vi "SetVolume.vi"(0 "reference in":refnum<class "MusicDevice.lvclass">, 2 "Volume":u8 max=100, 5 "Error In":errorcluster) -> (14 "reference out":refnum<class "MusicDevice.lvclass">, 19 "Error Out":errorcluster)   [LabVIEW 2024, in "MusicDevice.lvclass"]
uses:
  MusicDevice.lvclass
  MusicDevice.lvclass/MusicDevice.ctl
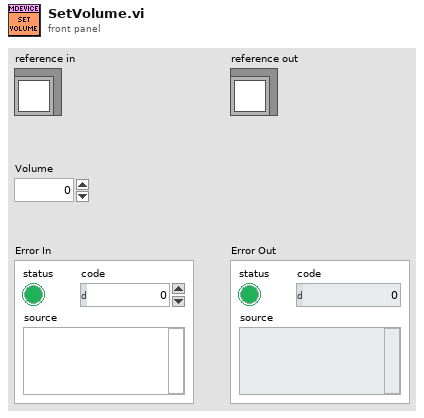
[diagram p1: front panel]
types:
  T1 = typedef "MusicDevice.lvclass/ObjectAttributes.ctl" = cluster{"State":bool, "Volume":u8}
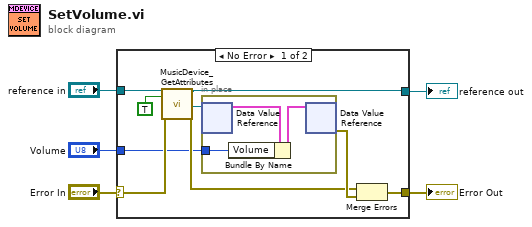
[diagram p0: block diagram]
diagram:
  n1 = case shown="No Error" "Error In" {
    selector: "Error In" -> [w14 w19]
    tunnel: [w11 w19] -> w4
    tunnel: [w9 w18] -> w2
    tunnel: "reference in" -> [w10 w18]
    tunnel: "Volume" -> [w6 _]
    frame No Error {
      n2 = call "MusicDevice_GetAttributes.vi"("reference in"=w10, "OnlyGetDvrReference(False)"=TRUE, "Error In"=w14) -> ("reference out"=w9:refnum<class "MusicDevice.lvclass">, "DataRef"=w7:refnum<data-value>, "Error Out"=w12:errorcluster)  [unwired: 13 in, 1 out]
      n3 = in-place {
        in-place-border: w6 -> [w17]
        n4 = in-place-dvr #1(w7) -> (w16:T1)  [unwired: 1 out]
        n5 = Bundle By Name(cluster=w16, "Volume"=w17) -> (w15:T1)
        n6 = in-place-dvr #1(w15) -> (w13:errorcluster)  [unwired: 1 out]
      }
      n7 = Merge Errors(w12, w13) -> (w11:errorcluster)
    }
    frame Error {
    }
  }
  "Error Out" <- w4
  "reference out" <- w2
